vi "Timer.vi"(8 "error in":errorcluster, 10 "limit":dbl, 11 "timer state":T1) -> (0 "error out":errorcluster, 2 "limit out":bool, 3 "elapsed":dbl)   [LabVIEW 2015]
uses:
  controls/timer state.ctl
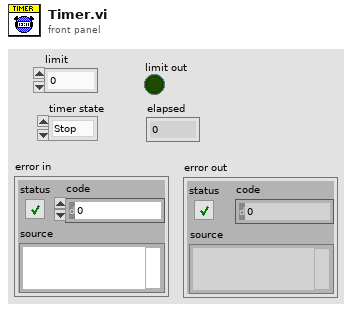
[diagram p1: front panel]
types:
  T1 = typedef "timer state.ctl" = enum16{"Stop", "Pause", "Start"}
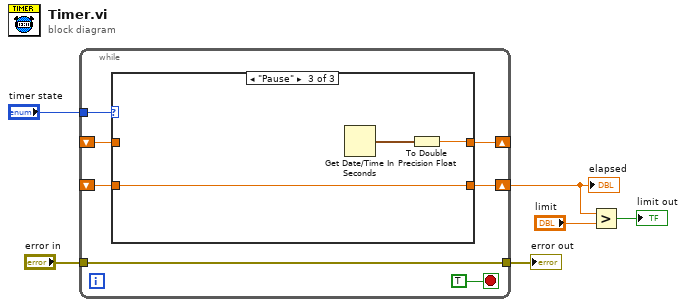
[diagram p0: block diagram]
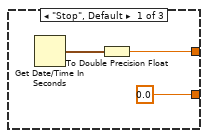
[diagram p2: hidden frame]
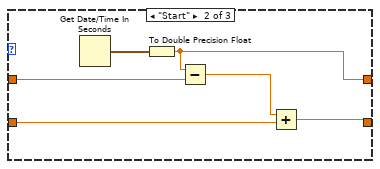
[diagram p3: hidden frame]
diagram:
  n1 = while {
    tunnel: "timer state" -> [w12]
    shift-right: [w11] -> _
    shift-left: _ -> [w9]
    shift-right: [w10] -> w5
    shift-left: _ -> [w8]
    tunnel: "error in" -> [w7]
    tunnel: [w7] -> w1
    stop <- TRUE stop-if-true
    n2 = case shown="\"Pause\"" w12 {
      tunnel: [w15 w20 w23] -> w11
      tunnel: [0.0 w17 w25] -> w10
      tunnel: w9 -> [_ w21 _]
      tunnel: w8 -> [_ w18 w25]
      frame "Stop", Default {
        n3 = Get Date/Time In Seconds() -> (seconds since 1Jan1904=w16:timestamp)
        n4 = To Double Precision Float(number=w16) -> (double precision float=w15:dbl)
      }
      frame "Start" {
        n5 = Get Date/Time In Seconds() -> (seconds since 1Jan1904=w22:timestamp)
        n6 = To Double Precision Float(number=w22) -> (double precision float=w20:dbl)
        n7 = Subtract(x=w20, y=w21) -> (x-y=w19:dbl)
        n8 = Add(x=w19, y=w18) -> (x+y=w17:dbl)
      }
      frame "Pause" {
        n9 = Get Date/Time In Seconds() -> (seconds since 1Jan1904=w24:timestamp)
        n10 = To Double Precision Float(number=w24) -> (double precision float=w23:dbl)
      }
    }
  }
  "elapsed" <- w5
  "error out" <- w1
  n11 = Greater?(x=w5, y="limit") -> (0:→"limit out":bool)
